vi "Revision Query.vi"(8 "error in (no error)":errorcluster, 11 "VISA resource name":refnum<visa-resource-name>) -> (0 "error out":errorcluster, 1 "Instrument Firmware Revision":string, 2 "Instrument Driver Revision":string, 3 "VISA resource name out":refnum<visa-resource-name>)   [LabVIEW 2019, in "Yokogawa WT300 Series.lvlib"]
doc: "Queries the current instrument firmware revision and instrument driver revision.\n\nFor detailed driver information including modification history, refer to the Readme file."
uses:
  Yokogawa WT300 Series.lvlib
panel:
  out "Error Count":i32
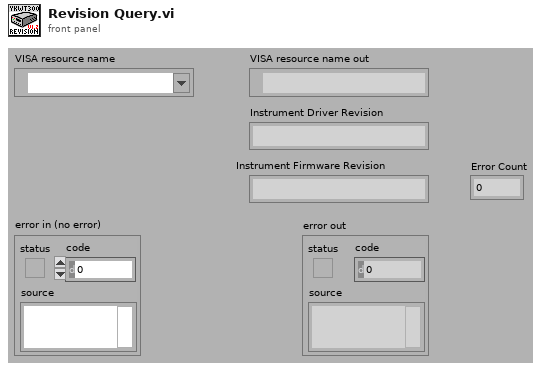
[diagram p1: front panel]
types:
  T1 = enum32{"invalid app kind", "Development System", "Run Time System", "Student Edition", "Embedded LabVIEW", "Evaluation", "Custom"}
  T2 = cluster{"Major":u16, "Minor":u16, "Fix":u16, "Build":u16}
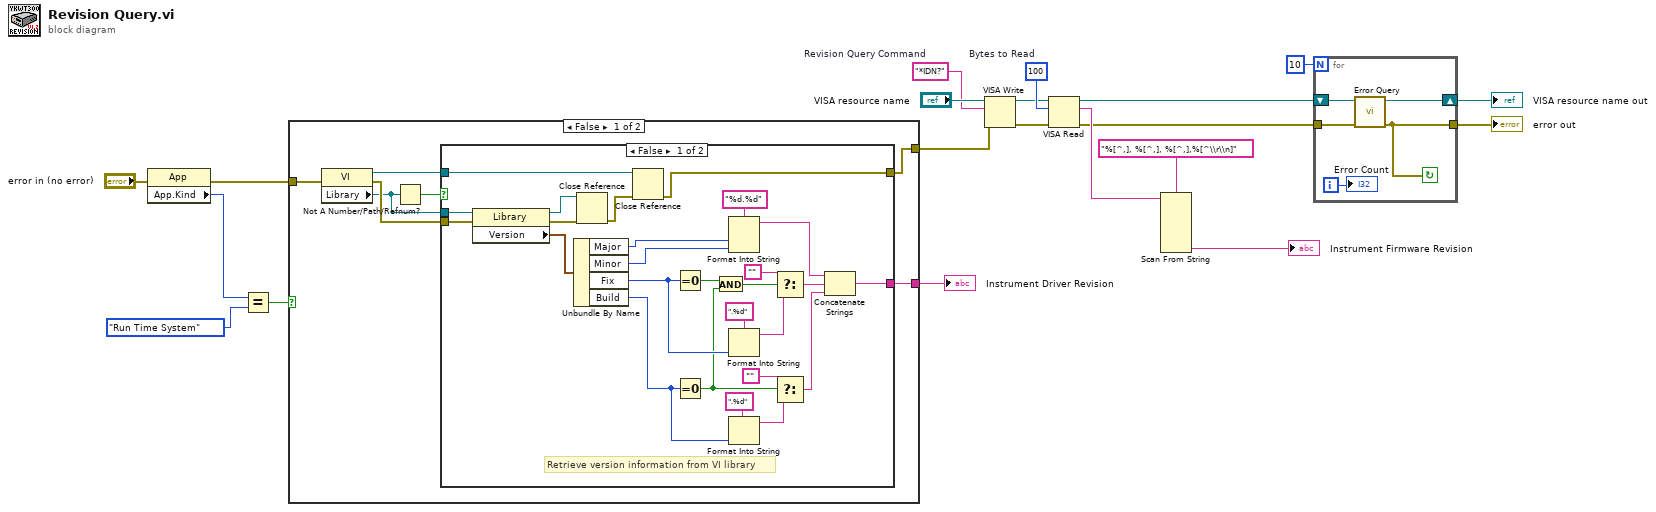
[diagram p0: block diagram]
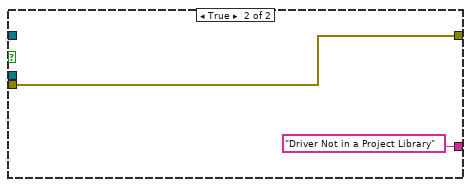
[diagram p2: hidden frame]
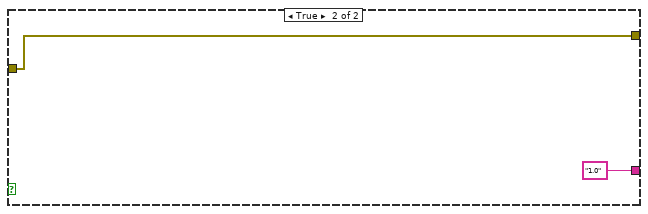
[diagram p3: hidden frame]
diagram:
  w15 = "*IDN?"  # Revision Query Command
  w18 = u32 100  # Bytes to Read
  n1 = property class="App"(error in="error in (no error)") -> (error out=w2:errorcluster, "App.Kind"=w5:T1)  [unwired: 1 in, 1 out]
  n2 = Equal?(x=w5, y=T1."Run Time System" ("アプリケーション: 種類")) -> (x = y?=w6:bool)
  n3 = case shown="False" w6 {
    tunnel: [w23 "1.0"] -> w8
    tunnel: w2 -> [w22 w56]
    tunnel: [w21 w56] -> w7
    frame False {
      n4 = property class="VI"(error in=w22) -> (reference out=w27:refnum<vi>, error out=w26:errorcluster, "Library"=w25:refnum<vi>)  [unwired: 1 in]
      n5 = Not A Number/Path/Refnum?(number/path/refnum=w25) -> (NaN/Path/Refnum?=w24:bool)
      n6 = case shown="False" w24 {
        tunnel: w27 -> [w50 _]
        tunnel: w26 -> [w35 w55]
        tunnel: [w30 w55] -> w21
        tunnel: [w29 "Driver Not in a Project Library"] -> w23
        tunnel: w25 -> [w28 _]
        frame False {
          # "Retrieve version information from VI library"
          n7 = property class="Library"(reference=w28, error in=w35) -> (reference out=w52:refnum<vi>, error out=w53:errorcluster, "Version"=w49:T2)
          n8 = Unbundle By Name(w49) -> ("Major"=w38:u16, "Minor"=w37:u16, "Fix"=w34:u16, "Build"=w36:u16)
          n9 = Close Reference(reference=w52, error in (no error)=w53) -> (error out=w51:errorcluster)
          n10 = Close Reference(reference=w50, error in (no error)=w51) -> (error out=w30:errorcluster)
          n11 = Equal To 0?(x=w34) -> (x = 0?=w33:bool)
          n12 = Equal To 0?(x=w36) -> (x = 0?=w32:bool)
          n13 = And(x=w33, y=w32) -> (x .and. y?=w31:bool)
          n14 = Format Into String(format string="%d.%d", w38, w37) -> (resulting string=w44:string)  [unwired: 2 in, 1 out]
          n15 = Format Into String(format string=".%d", w34) -> (resulting string=w46:string)  [unwired: 2 in, 1 out]
          n16 = Format Into String(format string=".%d", w36) -> (resulting string=w42:string)  [unwired: 2 in, 1 out]
          n17 = Select(t="", s=w31, f=w46) -> (s? t:f=w43:string)
          n18 = Select(t="", s=w32, f=w42) -> (s? t:f=w39:string)
          n19 = Concatenate Strings(w44, w43, w39) -> (w29:string)
        }
        frame True {
        }
      }
    }
    frame True {
    }
  }
  "Instrument Driver Revision" <- w8
  n20 = VISA Write(VISA resource name="VISA resource name", write buffer=w15, error in (no error)=w7) -> (VISA resource name out=w17:refnum<visa-resource-name>, error out=w16:errorcluster)  [unwired: 1 out]
  n21 = VISA Read(VISA resource name=w17, byte count=w18, error in (no error)=w16) -> (VISA resource name out=w11:refnum<visa-resource-name>, read buffer=w14:string, error out=w12:errorcluster)  [unwired: 1 out]
  n22 = Scan From String(format string="%[^,], %[^,], %[^,],%[^\\r\\n]", input string=w14) -> (output 4=→"Instrument Firmware Revision":string)  [unwired: 9 in, 3 out]
  n23 = for {
    N: 10 -> [_]
    shift-right: [w60] -> w10
    shift-left: w11 -> [w61]
    tunnel: w12 -> [w62]
    tunnel: [w59] -> w9
    i -> [w58]
    stop <- w59 continue-if-true
    n24 = call "Error Query.vi"("error in (no error)"=w62, "VISA resource name"=w61) -> ("error out"=w59:errorcluster, "VISA resource name out"=w60:refnum<visa-resource-name>)  [unwired: 6 in, 2 out]
    "Error Count" <- w58
  }
  "VISA resource name out" <- w10
  "error out" <- w9
